vi "Math_1_Term_API_Hierarchy.vi"   [LabVIEW 2021]
uses:
  Support/Function/One Terminal/SGL/AbsFunc_One Term_SGL.lvclass
  Support/Function/One Terminal/DBL/AbsFunc_One Term_DBL.lvclass
  Support/Function/One Terminal/EXT/AbsFunc_One Term_EXT.lvclass
  Support/Function/One Terminal/Cmplx SGL/AbsFunc_One Term_Complex SGL.lvclass
  Support/Function/One Terminal/Cmplx DBL/AbsFunc_One Term_Complex DBL.lvclass
  Support/Function/One Terminal/Cmplx EXT/AbsFunc_One Term_Complex EXT.lvclass
  Support/Function/One Terminal/I8/AbsFunc_One Term_I8.lvclass
  Support/Function/One Terminal/I16/AbsFunc_One Term_I16.lvclass
  Support/Function/One Terminal/I32/AbsFunc_One Term_I32.lvclass
  Support/Function/One Terminal/I64/AbsFunc_One Term_I64.lvclass
  Support/Function/One Terminal/U8/AbsFunc_One Term_U8.lvclass
  Support/Function/One Terminal/U16/AbsFunc_One Term_U16.lvclass
  Support/Function/One Terminal/U32/AbsFunc_One Term_U32.lvclass
  Support/Function/One Terminal/U64/AbsFunc_One Term_U64.lvclass
  Support/Function/One Terminal/Time/AbsFunc_One Term_Time.lvclass
  Support/Function/One Terminal/WFM_Numeric/AbsFunc_One Term_WFM_Numeric.lvclass
  Abs_Types/Double Float/Abs_Double Float.lvclass
  Support/Invert/DBL/Invert_DBL.lvclass
  Support/Increment/DBL/Increment_DBL.lvclass
  Support/Decrement/DBL/Decrement_DBL.lvclass
  Support/Decrement/SGL/Decrement_SGL.lvclass
  Support/Decrement/EXT/Decrement_EXT.lvclass
  Support/Decrement/CPLX_SGL/Decrement_CPLX_SGL.lvclass
  Support/Decrement/CPLX_DBL/Decrement_CPLX_DBL.lvclass
  Support/Decrement/CPLX_EXT/Decrement_CPLX_EXT.lvclass
  Support/Decrement/I8/Decrement_I8.lvclass
  Support/Decrement/I16/Decrement_I16.lvclass
  Support/Decrement/I32/Decrement_I32.lvclass
  Support/Decrement/I64/Decrement_I64.lvclass
  Support/Decrement/U8/Decrement_U8.lvclass
  Support/Decrement/U16/Decrement_U16.lvclass
  Support/Decrement/U32/Decrement_U32.lvclass
  Support/Decrement/U64/Decrement_U64.lvclass
  Support/Increment/SGL/Increment_SGL.lvclass
  Support/Increment/EXT/Increment_EXT.lvclass
  Support/Increment/CPLX_SGL/Increment_CPLX_SGL.lvclass
  Support/Increment/CPLX_DBL/Increment_CPLX_DBL.lvclass
  Support/Increment/CPLX_EXT/Increment_CPLX_EXT.lvclass
  Support/Increment/I8/Increment_I8.lvclass
  Support/Increment/I16/Increment_I16.lvclass
  Support/Increment/I32/Increment_I32.lvclass
  Support/Increment/I64/Increment_I64.lvclass
  Support/Increment/U8/Increment_U8.lvclass
  Support/Increment/U16/Increment_U16.lvclass
  Support/Increment/U32/Increment_U32.lvclass
  Support/Increment/U64/Increment_U64.lvclass
  Support/Increment/Time/Increment_Time.lvclass
  Support/Increment/WFM/Increment_WFM.lvclass
  Support/Invert/SGL/Invert_SGL.lvclass
  Support/Invert/EXT/Invert_EXT.lvclass
  Support/Invert/CPLX_SGL/Invert_CPLX_SGL.lvclass
  Support/Invert/CPLX_DBL/Invert_CPLX_DBL.lvclass
  Support/Invert/CPLX_EXT/Invert_CPLX_EXT.lvclass
  Support/Invert/I8/Invert_I8.lvclass
  Support/Invert/I16/Invert_I16.lvclass
  Support/Invert/I32/Invert_I32.lvclass
  Support/Invert/I64/Invert_I64.lvclass
  Support/Invert/WFM/Invert_WFM.lvclass
  Support/Reciprocal/SGL/Reciprocal_SGL.lvclass
  Support/Reciprocal/DBL/Reciprocal_DBL.lvclass
  Support/Reciprocal/EXT/Reciprocal_EXT.lvclass
  Support/Reciprocal/CPLX_DBL/Reciprocal_CPLX_DBL.lvclass
  Support/Reciprocal/CPLX_EXT/Reciprocal_CPLX_EXT.lvclass
  Support/Reciprocal/CPLX_SGL/Reciprocal_CPLX_SGL.lvclass
  Support/Reciprocal/Numeric/Reciprocal_Numeric.lvclass
panel:
  # "SEE DIAGRAM\nFOR Hierarchy"
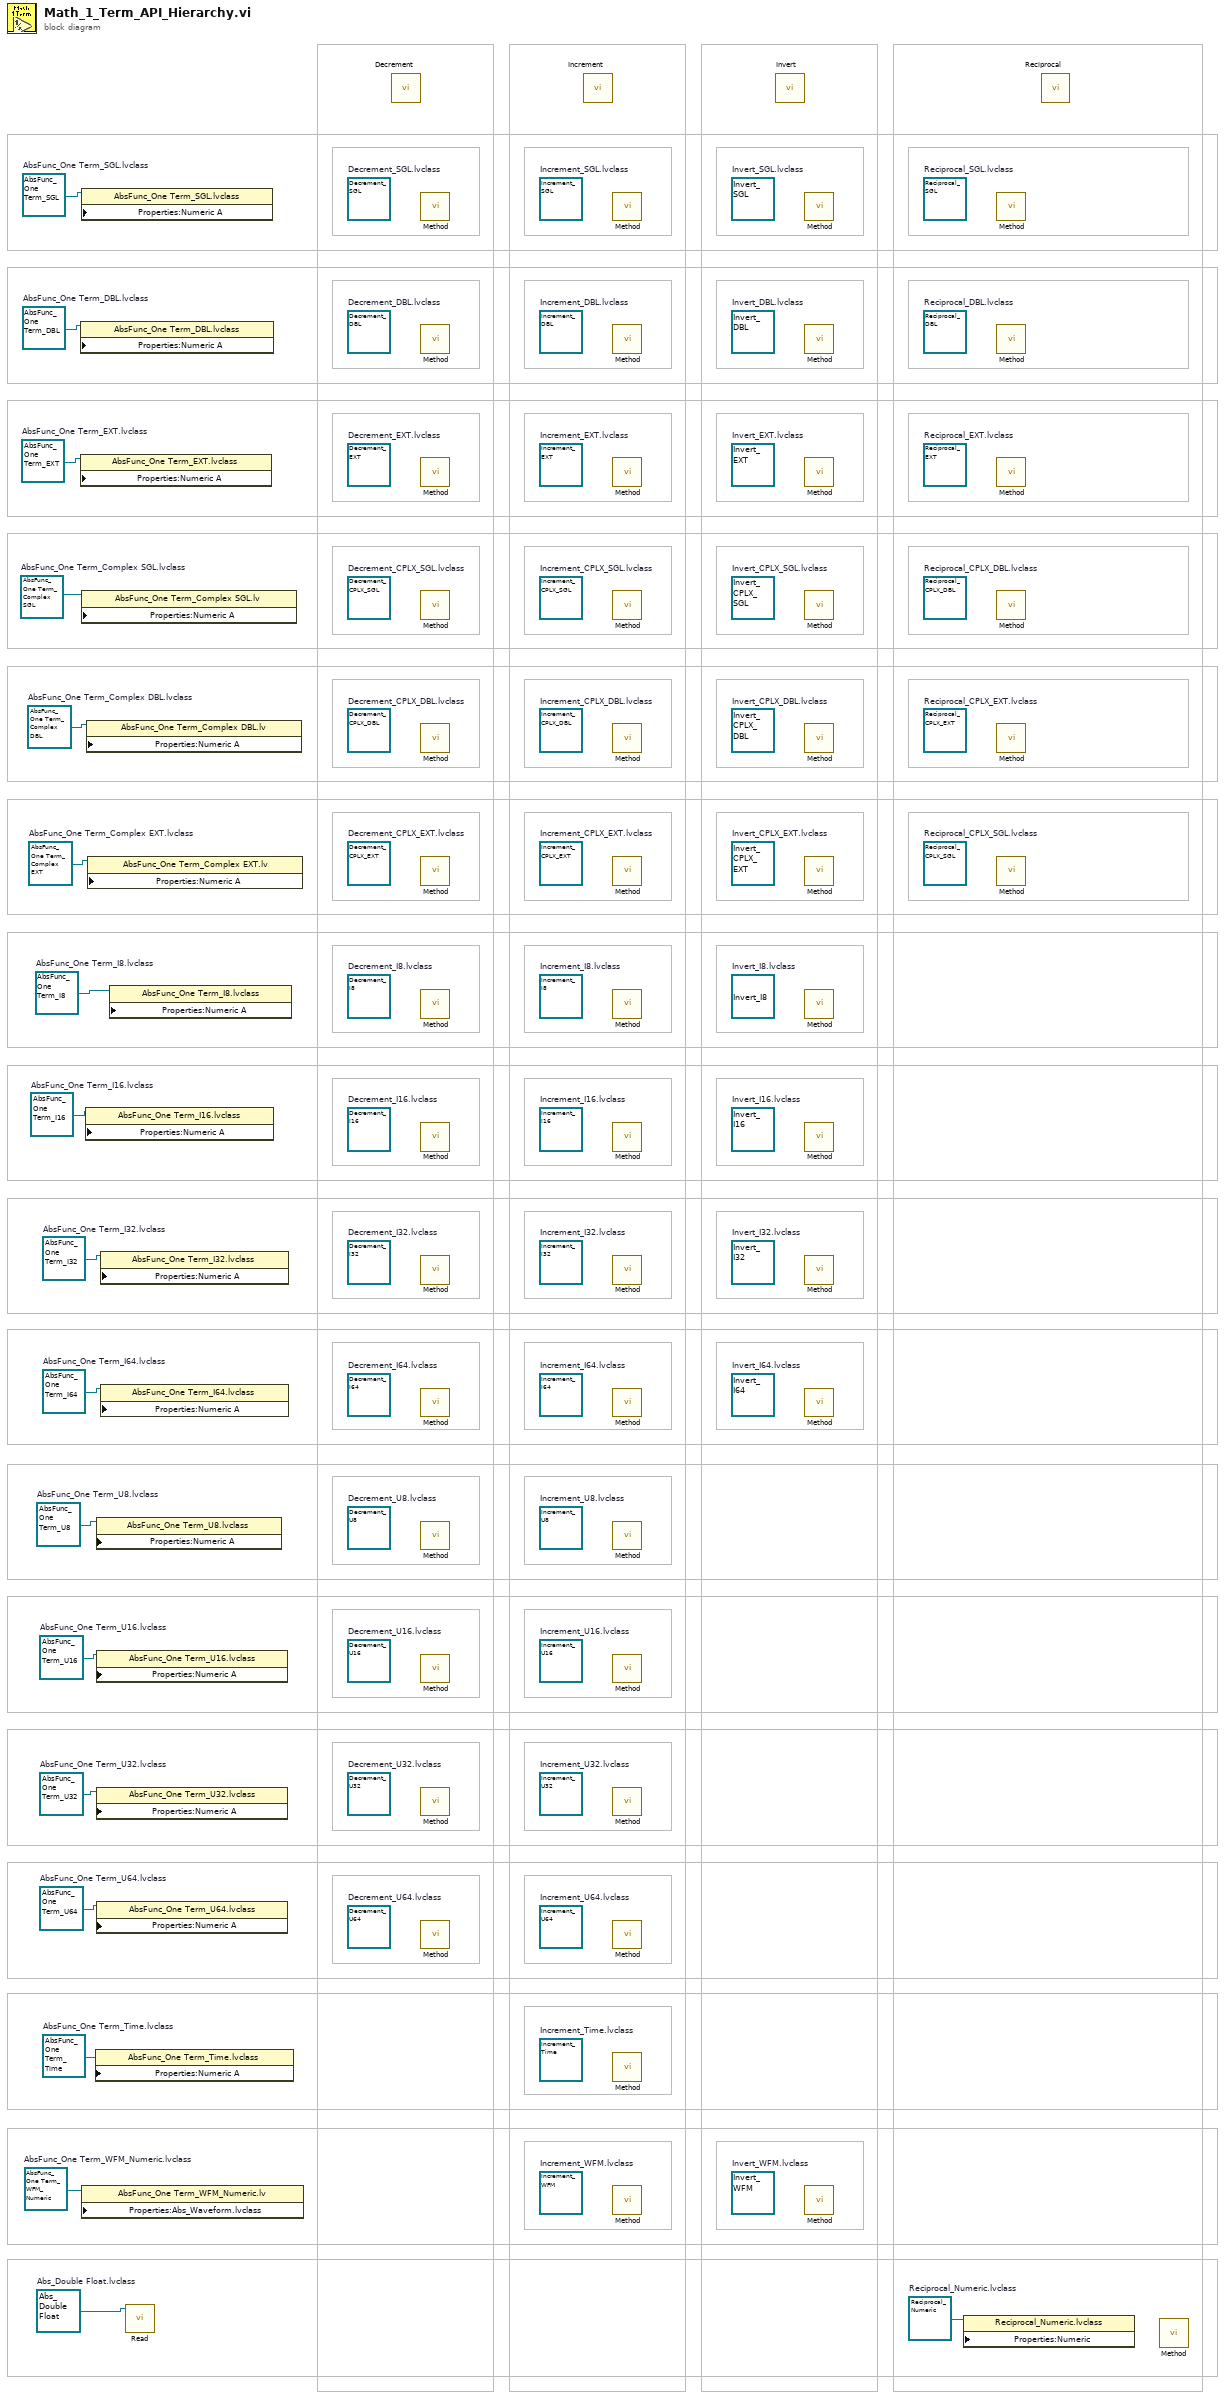
[diagram p0: block diagram]
diagram:
  w1 = refnum<class "Reciprocal_Numeric.lvclass"> refnum  # Reciprocal_Numeric.lvclass
  (unwired) refnum<class "Reciprocal_CPLX_SGL.lvclass"> refnum  # Reciprocal_CPLX_SGL.lvclass
  (unwired) refnum<class "Reciprocal_CPLX_EXT.lvclass"> refnum  # Reciprocal_CPLX_EXT.lvclass
  (unwired) refnum<class "Reciprocal_CPLX_DBL.lvclass"> refnum  # Reciprocal_CPLX_DBL.lvclass
  (unwired) refnum<class "Reciprocal_EXT.lvclass"> refnum  # Reciprocal_EXT.lvclass
  (unwired) refnum<class "Reciprocal_DBL.lvclass"> refnum  # Reciprocal_DBL.lvclass
  (unwired) refnum<class "Reciprocal_SGL.lvclass"> refnum  # Reciprocal_SGL.lvclass
  (unwired) refnum<class "Invert_WFM.lvclass"> refnum  # Invert_WFM.lvclass
  (unwired) refnum<class "Invert_I64.lvclass"> refnum  # Invert_I64.lvclass
  (unwired) refnum<class "Invert_I32.lvclass"> refnum  # Invert_I32.lvclass
  (unwired) refnum<class "Invert_I16.lvclass"> refnum  # Invert_I16.lvclass
  (unwired) refnum<class "Invert_I8.lvclass"> refnum  # Invert_I8.lvclass
  (unwired) refnum<class "Invert_CPLX_EXT.lvclass"> refnum  # Invert_CPLX_EXT.lvclass
  (unwired) refnum<class "Invert_CPLX_DBL.lvclass"> refnum  # Invert_CPLX_DBL.lvclass
  (unwired) refnum<class "Invert_CPLX_SGL.lvclass"> refnum  # Invert_CPLX_SGL.lvclass
  (unwired) refnum<class "Invert_EXT.lvclass"> refnum  # Invert_EXT.lvclass
  (unwired) refnum<class "Invert_DBL.lvclass"> refnum  # Invert_DBL.lvclass
  (unwired) refnum<class "Invert_SGL.lvclass"> refnum  # Invert_SGL.lvclass
  (unwired) refnum<class "Increment_WFM.lvclass"> refnum  # Increment_WFM.lvclass
  (unwired) refnum<class "Increment_Time.lvclass"> refnum  # Increment_Time.lvclass
  (unwired) refnum<class "Increment_U64.lvclass"> refnum  # Increment_U64.lvclass
  (unwired) refnum<class "Increment_U32.lvclass"> refnum  # Increment_U32.lvclass
  (unwired) refnum<class "Increment_U16.lvclass"> refnum  # Increment_U16.lvclass
  (unwired) refnum<class "Increment_U8.lvclass"> refnum  # Increment_U8.lvclass
  (unwired) refnum<class "Increment_I64.lvclass"> refnum  # Increment_I64.lvclass
  (unwired) refnum<class "Increment_I32.lvclass"> refnum  # Increment_I32.lvclass
  (unwired) refnum<class "Increment_I16.lvclass"> refnum  # Increment_I16.lvclass
  (unwired) refnum<class "Increment_I8.lvclass"> refnum  # Increment_I8.lvclass
  (unwired) refnum<class "Increment_CPLX_EXT.lvclass"> refnum  # Increment_CPLX_EXT.lvclass
  (unwired) refnum<class "Increment_CPLX_DBL.lvclass"> refnum  # Increment_CPLX_DBL.lvclass
  (unwired) refnum<class "Increment_CPLX_SGL.lvclass"> refnum  # Increment_CPLX_SGL.lvclass
  (unwired) refnum<class "Increment_EXT.lvclass"> refnum  # Increment_EXT.lvclass
  (unwired) refnum<class "Increment_DBL.lvclass"> refnum  # Increment_DBL.lvclass
  (unwired) refnum<class "Increment_SGL.lvclass"> refnum  # Increment_SGL.lvclass
  (unwired) refnum<class "Decrement_U64.lvclass"> refnum  # Decrement_U64.lvclass
  (unwired) refnum<class "Decrement_U32.lvclass"> refnum  # Decrement_U32.lvclass
  (unwired) refnum<class "Decrement_U16.lvclass"> refnum  # Decrement_U16.lvclass
  (unwired) refnum<class "Decrement_U8.lvclass"> refnum  # Decrement_U8.lvclass
  (unwired) refnum<class "Decrement_I64.lvclass"> refnum  # Decrement_I64.lvclass
  (unwired) refnum<class "Decrement_I32.lvclass"> refnum  # Decrement_I32.lvclass
  (unwired) refnum<class "Decrement_I16.lvclass"> refnum  # Decrement_I16.lvclass
  (unwired) refnum<class "Decrement_I8.lvclass"> refnum  # Decrement_I8.lvclass
  (unwired) refnum<class "Decrement_CPLX_EXT.lvclass"> refnum  # Decrement_CPLX_EXT.lvclass
  (unwired) refnum<class "Decrement_CPLX_DBL.lvclass"> refnum  # Decrement_CPLX_DBL.lvclass
  (unwired) refnum<class "Decrement_CPLX_SGL.lvclass"> refnum  # Decrement_CPLX_SGL.lvclass
  (unwired) refnum<class "Decrement_EXT.lvclass"> refnum  # Decrement_EXT.lvclass
  (unwired) refnum<class "Decrement_DBL.lvclass"> refnum  # Decrement_DBL.lvclass
  (unwired) refnum<class "Decrement_SGL.lvclass"> refnum  # Decrement_SGL.lvclass
  w2 = refnum<class "Abs_Double Float.lvclass"> refnum  # Abs_Double Float.lvclass
  w3 = refnum<class "AbsFunc_One Term_WFM_Numeric.lvclass"> refnum  # AbsFunc_One Term_WFM_Numeric.lvclass
  w4 = refnum<class "AbsFunc_One Term_Time.lvclass"> refnum  # AbsFunc_One Term_Time.lvclass
  w6 = refnum<class "AbsFunc_One Term_U64.lvclass"> refnum  # AbsFunc_One Term_U64.lvclass
  w5 = refnum<class "AbsFunc_One Term_U32.lvclass"> refnum  # AbsFunc_One Term_U32.lvclass
  w7 = refnum<class "AbsFunc_One Term_U16.lvclass"> refnum  # AbsFunc_One Term_U16.lvclass
  w8 = refnum<class "AbsFunc_One Term_U8.lvclass"> refnum  # AbsFunc_One Term_U8.lvclass
  w9 = refnum<class "AbsFunc_One Term_I64.lvclass"> refnum  # AbsFunc_One Term_I64.lvclass
  w10 = refnum<class "AbsFunc_One Term_I32.lvclass"> refnum  # AbsFunc_One Term_I32.lvclass
  w11 = refnum<class "AbsFunc_One Term_I16.lvclass"> refnum  # AbsFunc_One Term_I16.lvclass
  w12 = refnum<class "AbsFunc_One Term_I8.lvclass"> refnum  # AbsFunc_One Term_I8.lvclass
  w13 = refnum<class "AbsFunc_One Term_Complex EXT.lvclass"> refnum  # AbsFunc_One Term_Complex EXT.lvclass
  w14 = refnum<class "AbsFunc_One Term_Complex DBL.lvclass"> refnum  # AbsFunc_One Term_Complex DBL.lvclass
  w15 = refnum<class "AbsFunc_One Term_Complex SGL.lvclass"> refnum  # AbsFunc_One Term_Complex SGL.lvclass
  w16 = refnum<class "AbsFunc_One Term_EXT.lvclass"> refnum  # AbsFunc_One Term_EXT.lvclass
  w17 = refnum<class "AbsFunc_One Term_DBL.lvclass"> refnum  # AbsFunc_One Term_DBL.lvclass
  w18 = refnum<class "AbsFunc_One Term_SGL.lvclass"> refnum  # AbsFunc_One Term_SGL.lvclass
  n1 = property class="AbsFunc_One Term_DBL.lvclass" props=["Properties:Numeric A"](reference=w17) -> ()  [unwired: 2 in, 2 out]
  n2 = property class="AbsFunc_One Term_EXT.lvclass" props=["Properties:Numeric A"](reference=w16) -> ()  [unwired: 2 in, 2 out]
  n3 = property class="AbsFunc_One Term_SGL.lvclass" props=["Properties:Numeric A"](reference=w18) -> ()  [unwired: 2 in, 2 out]
  n4 = property class="AbsFunc_One Term_Complex SGL.lv" props=["Properties:Numeric A"](reference=w15) -> ()  [unwired: 2 in, 2 out]
  n5 = property class="AbsFunc_One Term_WFM_Numeric.lv" props=["Properties:Abs_Waveform.lvclass"](reference=w3) -> ()  [unwired: 2 in, 2 out]
  n6 = property class="AbsFunc_One Term_I16.lvclass" props=["Properties:Numeric A"](reference=w11) -> ()  [unwired: 2 in, 2 out]
  n7 = property class="AbsFunc_One Term_Complex DBL.lv" props=["Properties:Numeric A"](reference=w14) -> ()  [unwired: 2 in, 2 out]
  n8 = property class="AbsFunc_One Term_Complex EXT.lv" props=["Properties:Numeric A"](reference=w13) -> ()  [unwired: 2 in, 2 out]
  n9 = property class="AbsFunc_One Term_Time.lvclass" props=["Properties:Numeric A"](reference=w4) -> ()  [unwired: 2 in, 2 out]
  n10 = property class="AbsFunc_One Term_U8.lvclass" props=["Properties:Numeric A"](reference=w8) -> ()  [unwired: 2 in, 2 out]
  n11 = property class="AbsFunc_One Term_U16.lvclass" props=["Properties:Numeric A"](reference=w7) -> ()  [unwired: 2 in, 2 out]
  n12 = property class="AbsFunc_One Term_U32.lvclass" props=["Properties:Numeric A"](reference=w5) -> ()  [unwired: 2 in, 2 out]
  n13 = property class="AbsFunc_One Term_U64.lvclass" props=["Properties:Numeric A"](reference=w6) -> ()  [unwired: 2 in, 2 out]
  n14 = property class="AbsFunc_One Term_I32.lvclass" props=["Properties:Numeric A"](reference=w10) -> ()  [unwired: 2 in, 2 out]
  n15 = property class="AbsFunc_One Term_I64.lvclass" props=["Properties:Numeric A"](reference=w9) -> ()  [unwired: 2 in, 2 out]
  n16 = property class="AbsFunc_One Term_I8.lvclass" props=["Properties:Numeric A"](reference=w12) -> ()  [unwired: 2 in, 2 out]
  n17 = call-dynamic "Read.vi"("Double Float.lvclass_340760 in"=w2) -> ()  [unwired: 8 in, 3 out]
  n18 = call-poly "Decrement.vi"() -> ()  [unwired: 5 in, 1 out]
  n19 = call "Method.vi"() -> ()  [unwired: 5 in, 1 out]
  n20 = call "Method.vi"() -> ()  [unwired: 5 in, 1 out]
  n21 = call "Method.vi"() -> ()  [unwired: 5 in, 1 out]
  n22 = call "Method.vi"() -> ()  [unwired: 5 in, 1 out]
  n23 = call "Method.vi"() -> ()  [unwired: 5 in, 1 out]
  n24 = call "Method.vi"() -> ()  [unwired: 5 in, 1 out]
  n25 = call "Method.vi"() -> ()  [unwired: 5 in, 1 out]
  n26 = call "Method.vi"() -> ()  [unwired: 5 in, 1 out]
  n27 = call "Method.vi"() -> ()  [unwired: 5 in, 1 out]
  n28 = call "Method.vi"() -> ()  [unwired: 5 in, 1 out]
  n29 = call "Method.vi"() -> ()  [unwired: 5 in, 1 out]
  n30 = call "Method.vi"() -> ()  [unwired: 5 in, 1 out]
  n31 = call "Method.vi"() -> ()  [unwired: 5 in, 1 out]
  n32 = call "Method.vi"() -> ()  [unwired: 5 in, 1 out]
  n33 = call-poly "Increment.vi"() -> ()  [unwired: 5 in, 1 out]
  n34 = call "Method.vi"() -> ()  [unwired: 5 in, 1 out]
  n35 = call "Method.vi"() -> ()  [unwired: 5 in, 1 out]
  n36 = call "Method.vi"() -> ()  [unwired: 5 in, 1 out]
  n37 = call "Method.vi"() -> ()  [unwired: 5 in, 1 out]
  n38 = call "Method.vi"() -> ()  [unwired: 5 in, 1 out]
  n39 = call "Method.vi"() -> ()  [unwired: 5 in, 1 out]
  n40 = call "Method.vi"() -> ()  [unwired: 5 in, 1 out]
  n41 = call "Method.vi"() -> ()  [unwired: 5 in, 1 out]
  n42 = call "Method.vi"() -> ()  [unwired: 5 in, 1 out]
  n43 = call "Method.vi"() -> ()  [unwired: 5 in, 1 out]
  n44 = call "Method.vi"() -> ()  [unwired: 5 in, 1 out]
  n45 = call "Method.vi"() -> ()  [unwired: 5 in, 1 out]
  n46 = call "Method.vi"() -> ()  [unwired: 5 in, 1 out]
  n47 = call "Method.vi"() -> ()  [unwired: 5 in, 1 out]
  n48 = call "Method.vi"() -> ()  [unwired: 5 in, 1 out]
  n49 = call "Method.vi"() -> ()  [unwired: 5 in, 1 out]
  n50 = call-poly "Invert.vi"() -> ()  [unwired: 5 in, 1 out]
  n51 = call "Method.vi"() -> ()  [unwired: 5 in, 1 out]
  n52 = call "Method.vi"() -> ()  [unwired: 5 in, 1 out]
  n53 = call "Method.vi"() -> ()  [unwired: 5 in, 1 out]
  n54 = call "Method.vi"() -> ()  [unwired: 5 in, 1 out]
  n55 = call "Method.vi"() -> ()  [unwired: 5 in, 1 out]
  n56 = call "Method.vi"() -> ()  [unwired: 5 in, 1 out]
  n57 = call "Method.vi"() -> ()  [unwired: 5 in, 1 out]
  n58 = call "Method.vi"() -> ()  [unwired: 5 in, 1 out]
  n59 = call "Method.vi"() -> ()  [unwired: 5 in, 1 out]
  n60 = call "Method.vi"() -> ()  [unwired: 5 in, 1 out]
  n61 = call "Method.vi"() -> ()  [unwired: 5 in, 1 out]
  n62 = property class="Reciprocal_Numeric.lvclass" props=["Properties:Numeric"](reference=w1) -> ()  [unwired: 2 in, 2 out]
  n63 = call "Method.vi"() -> ()  [unwired: 5 in, 1 out]
  n64 = call "Method.vi"() -> ()  [unwired: 5 in, 1 out]
  n65 = call "Method.vi"() -> ()  [unwired: 5 in, 1 out]
  n66 = call "Method.vi"() -> ()  [unwired: 5 in, 1 out]
  n67 = call "Method.vi"() -> ()  [unwired: 5 in, 1 out]
  n68 = call "Method.vi"() -> ()  [unwired: 5 in, 1 out]
  n69 = call-poly "Reciprocal.vi"() -> ()  [unwired: 5 in, 1 out]
  n70 = call "Method.vi"() -> ()  [unwired: 5 in, 1 out]
